vi "LoadMotionPositions.vi"(7 "TestZT":cluster{"Z mm":dbl, "Horizontal T deg":dbl}, 8 "error in (no error)":errorcluster, 9 "Position Array":T1(array[cluster]), 11 "Sequence in":refnum<class "Sequence.lvclass">) -> (0 "error out":errorcluster, 3 "Sequence out":refnum<class "Sequence.lvclass">)   [LabVIEW 2018, in "Sequence.lvclass"]
doc: "insert XYXT coordinates into the test sequence for Park and Measure sequences only.\nInsert absolute values for Horizontal and Vertical."
uses:
  Sequence.lvclass
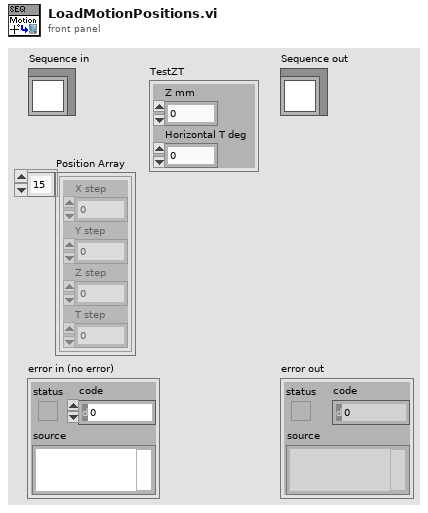
[diagram p1: front panel]
types:
  T1 = cluster{"X step":dbl, "Y step":dbl, "Z step":dbl, "T step":dbl}[]
  T2 = cluster{"X step":dbl, "Y step":dbl, "Z step":dbl, "T step":dbl}
  T3 = typedef "mWaveTestStep.ctl" = cluster{"StepType":T4, "RF In/Out":T5, "Module/Raster":i32, "Polarization":T6, "AO-64 Array":dbl[], "Position":T7[]}
  T4 = typedef "TestStepTypes.ctl" = enum16{"MotionFF-M2", "Motion", "SweepTest", "RasterTest", "Finish", "64ModuleCfg"}
  T5 = typedef "RF Direction.ctl" = enum16{"Tx - RF In", "Rx - RF Out"}
  T6 = typedef "PolarizationSelect.ctl" = enum16{"Vertical", "Horizontal"}
  T7 = typedef "singleAxisMoveDef.ctl" = cluster{"mmWave Axis":T8, "eng. value":dbl}
  T8 = typedef "mmWaveAxis.ctl" = string
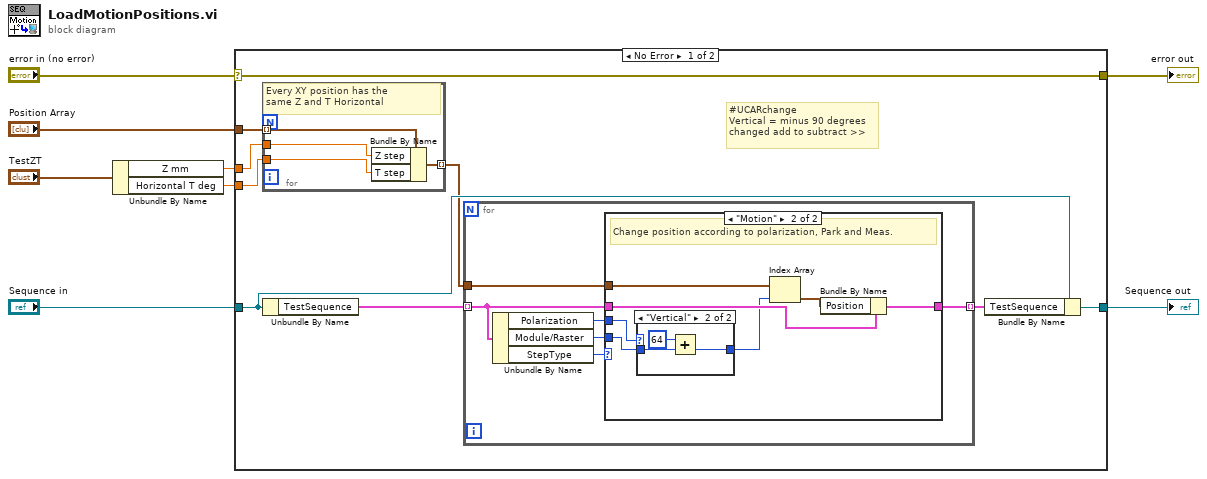
[diagram p0: block diagram]
diagram:
  n1 = Unbundle By Name("TestZT") -> ("Z mm"=w2:dbl, "Horizontal T deg"=w1:dbl)
  n2 = case shown="No Error" "error in (no error)" {
    selector: "error in (no error)" -> [w17 w41]
    tunnel: [w17 w41] -> w7
    tunnel: [w15 w40] -> w5
    tunnel: "Sequence in" -> [w16 w40]
    tunnel: "Position Array" -> [w12 _]
    tunnel: w2 -> [w10 _]
    tunnel: w1 -> [w9 _]
    frame No Error {
      # "#UCARchange \nVertical = minus 90 degrees\nchanged add to subtract >>"
      n3 = for {
        tunnel: [w20] -> w11 mode=indexing
        tunnel: w12 -> [w21] mode=indexing
        tunnel: w10 -> [w19]
        tunnel: w9 -> [w18]
        # "Every XY position has the\nsame Z and T Horizontal"
        n4 = Bundle By Name(cluster=w21, "Z step"=w19, "T step"=w18) -> (w20:T2)
      }
      n5 = Unbundle By Name(w16) -> ("TestSequence"=w14:T3[])
      n6 = for {
        tunnel: w14 -> [w23] mode=indexing
        tunnel: w11 -> [w24]
        tunnel: [w22] -> w13 mode=indexing
        n7 = Unbundle By Name(w23) -> ("Polarization"=w26:T6, "Module/Raster"=w25:i32, "StepType"=w27:T4)
        n8 = case shown="\"Motion\"" w27 {
          tunnel: w26 -> [_ w31]
          tunnel: w25 -> [_ w30]
          tunnel: w24 -> [_ w35]
          tunnel: [w28 w33] -> w22
          tunnel: w23 -> [w28 w34]
          frame "MotionFF-M2", Default {
          }
          frame "Motion" {
            # "Change position according to polarization, Park and Meas."
            n9 = case shown="\"Vertical\"" w31 {
              tunnel: [w36 w38] -> w29
              tunnel: w30 -> [w36 w39]
              frame "Horizontal" {
              }
              frame "Vertical" {
                n10 = Add(x=64, y=w39) -> (x+y=w38:i32)
              }
            }
            n11 = Index Array(array=w35, index=w29) -> (element=w32:T2)
            n12 = Bundle By Name(cluster=w34, "Position"=w32) -> (w33:T3)
          }
        }
      }
      n13 = Bundle By Name(cluster=w16, "TestSequence"=w13) -> (w15:refnum<class "Sequence.lvclass">)
    }
    frame Error {
    }
  }
  "error out" <- w7
  "Sequence out" <- w5
